vi "12版本XY图光标  随鼠标移动显示对应位置处数据.vi"() -> ()   [LabVIEW 2012]
panel:
  out "频率":string
  out "振动加速度":string
  in  "停止":bool
  out "XY图":cluster{dbl[], dbl[]}(graph)
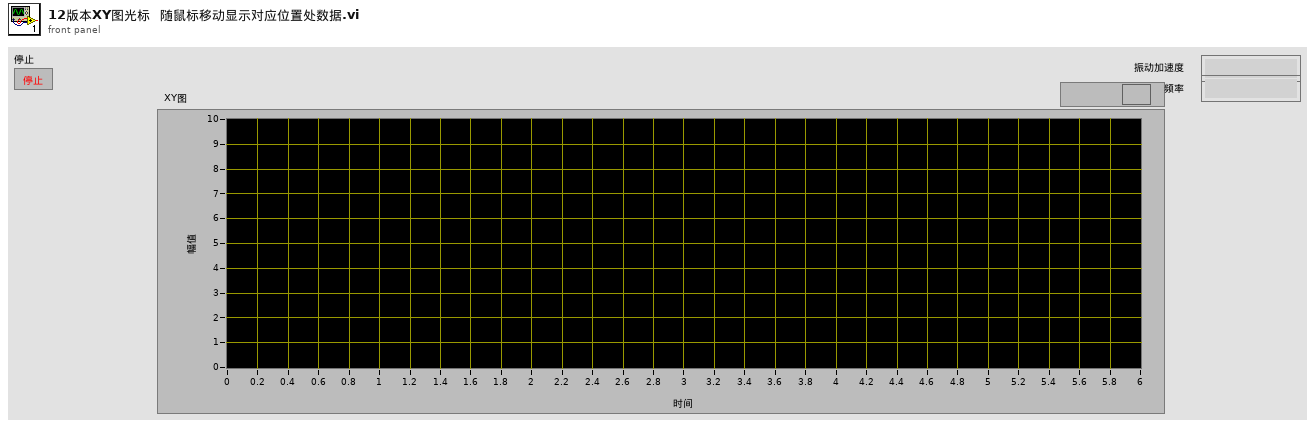
[diagram p1: front panel]
types:
  T1 = typedef "LVPoint32TypeDef.ctl" = cluster{"Horizontal":i32, "Vertical":i32}
  T2 = typedef "LVRectTypeDef.ctl" = cluster{"Left":i16, "Top":i16, "Right":i16, "Bottom":i16}
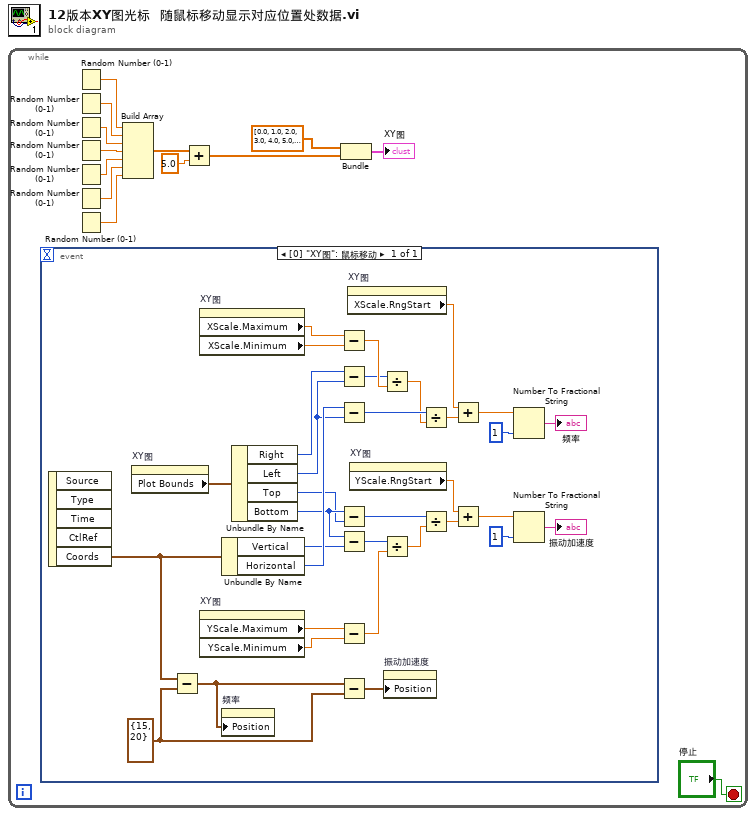
[diagram p0: block diagram]
diagram:
  n1 = while {
    stop <- "停止" stop-if-true
    n2 = event shown="[0] \"XY图\": 鼠标移动" {
      selector: _ -> [_]
      dyn-events: _ -> [_]
      timeout: _ -> [_]
      event "XY图": Mouse Move {
        w46 = cluster{"Horizontal":i32, "Vertical":i32} {"Horizontal"=15, "Vertical"=20} ("y")
        n3 = event-data() -> ("Coords"=w14:T1)  [unwired: 1 in, 4 out]
        n4 = property on="XY图" class="XYGraph (严格)"() -> ("Plot Bounds"=w42:T2)  [unwired: 2 in, 2 out]
        n5 = Subtract(x=w14, y=w46) -> (x-y=w17:T1)
        n6 = property on="XY图" class="XYGraph (严格)"() -> ("XScale.Maximum"=w44:dbl, "XScale.Minimum"=w43:dbl)  [unwired: 2 in, 2 out]
        n7 = property on="XY图" class="XYGraph (严格)"() -> ("YScale.Maximum"=w31:dbl, "YScale.Minimum"=w30:dbl)  [unwired: 2 in, 2 out]
        n8 = Unbundle By Name(w14) -> ("Vertical"=w27:i32, "Horizontal"=w40:i32)
        n9 = property on="频率" class="Str"("Position"=w17) -> ()  [unwired: 2 in, 2 out]
        n10 = Unbundle By Name(w42) -> ("Right"=w41:i16, "Left"=w39:i16, "Top"=w25:i16, "Bottom"=w26:i16)
        n11 = Subtract(x=w44, y=w43) -> (x-y=w38:dbl)
        n12 = Subtract(x=w41, y=w39) -> (x-y=w37:i16)
        n13 = Subtract(x=w40, y=w39) -> (x-y=w33:i32)
        n14 = Subtract(x=w26, y=w25) -> (x-y=w22:i16)
        n15 = Subtract(x=w26, y=w27) -> (x-y=w23:i32)
        n16 = Subtract(x=w31, y=w30) -> (x-y=w24:dbl)
        n17 = Subtract(x=w17, y=w46) -> (x-y=w45:T1)
        n18 = property on="XY图" class="XYGraph (严格)"() -> ("XScale.RngStart"=w36:dbl)  [unwired: 2 in, 2 out]
        n19 = property on="XY图" class="XYGraph (严格)"() -> ("YScale.RngStart"=w21:dbl)  [unwired: 2 in, 2 out]
        n20 = Divide(x=w37, y=w38) -> (x/y=w32:dbl)
        n21 = Divide(x=w23, y=w24) -> (x/y=w29:dbl)
        n22 = property on="振动加速度" class="Str"("Position"=w45) -> ()  [unwired: 2 in, 2 out]
        n23 = Divide(x=w33, y=w32) -> (x/y=w34:dbl)
        n24 = Divide(x=w22, y=w29) -> (x/y=w28:dbl)
        n25 = Add(x=w36, y=w34) -> (x+y=w35:dbl)
        n26 = Add(x=w21, y=w28) -> (x+y=w20:dbl)
        n27 = Number To Fractional String(number=w35, precision (6)=i16 1 ("精度(6)")) -> (F-format string=→"频率":string)  [unwired: 2 in]
        n28 = Number To Fractional String(number=w20, precision (6)=i16 1 ("精度(6)")) -> (F-format string=→"振动加速度":string)  [unwired: 2 in]
      }
    }
    n29 = Random Number (0-1)() -> (number: 0 to 1=w12:dbl)
    n30 = Random Number (0-1)() -> (number: 0 to 1=w11:dbl)
    n31 = Random Number (0-1)() -> (number: 0 to 1=w10:dbl)
    n32 = Random Number (0-1)() -> (number: 0 to 1=w9:dbl)
    n33 = Random Number (0-1)() -> (number: 0 to 1=w8:dbl)
    n34 = Random Number (0-1)() -> (number: 0 to 1=w7:dbl)
    n35 = Random Number (0-1)() -> (number: 0 to 1=w6:dbl)
    n36 = Build Array(w12, w11, w10, w9, w8, w7, w6) -> (w2:dbl[])
    n37 = Add(x=w2, y=5.0) -> (x+y=w1:dbl[])
    n38 = Bundle(dbl[] [0.0, 1.0, 2.0, 3.0, 4.0, 5.0, 6.0], w1) -> (→"XY图":cluster{dbl[], dbl[]})  [unwired: 1 in]
  }
